vi "Remove Chassis.vi"(0 "SLSC Local in":refnum<class "SLSC Local.lvclass">, 5 "chassis":refnum<k21>, 11 "error in (no error)":errorcluster) -> (4 "SLSC Local out":refnum<class "SLSC Local.lvclass">, 15 "error out":errorcluster)   [LabVIEW 2016, in "SLSC Interfaces.lvlib" / "SLSC Local.lvclass"]
uses:
  SLSC Local.lvclass
  C:/Users/tblair/Documents/SLSC-Interface/Source/SLSC Interface Class/SLSC Interface.lvclass
  <vilib>/SLSC/SLSC.lvlib
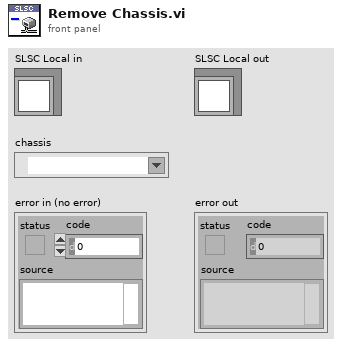
[diagram p1: front panel]
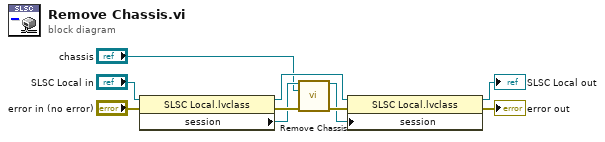
[diagram p0: block diagram]
diagram:
  n1 = property class="SLSC Local.lvclass"(reference="SLSC Local in", error in="error in (no error)") -> (reference out=w8:refnum<class "SLSC Local.lvclass">, error out=w10:errorcluster, "session"=w7:refnum<k21>)
  n2 = call <vilib>:"Remove Chassis.vi"("session in"=w7, "chassis"="chassis", "error in (no error)"=w10) -> ("session out"=w6:refnum<k21>, "error out"=w9:errorcluster)  [unwired: 11 in]
  n3 = property class="SLSC Local.lvclass"(reference=w8, error in=w9, "session"=w6) -> (reference out=→"SLSC Local out":refnum<class "SLSC Local.lvclass">, error out=→"error out":errorcluster)
